vi "IECal-Find Last N.vi"(0 "Data folder":path, 7 "Speaker":string) -> (4 "paths":path[](array[path]), 8 "names":string[](array[string]))   [LabVIEW 2020]
doc: "This helper VI plots all of the in ear calibration files in the current experiment data folder.\n\nKEH 9/10/09"
uses:
  <vilib>/regexp/Match Regular Expression.xnode
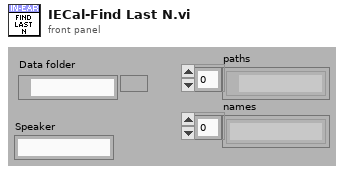
[diagram p1: front panel]
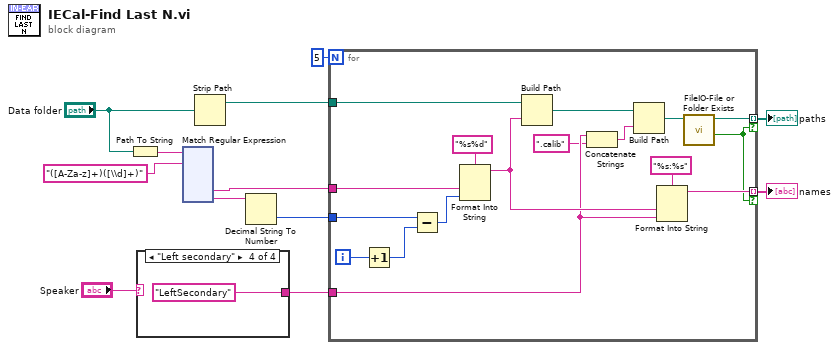
[diagram p0: block diagram]
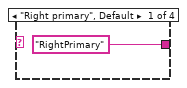
[diagram p2: hidden frame]
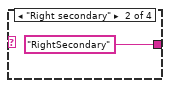
[diagram p3: hidden frame]
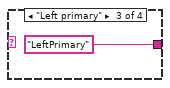
[diagram p4: hidden frame]
diagram:
  n1 = Path To String(path="Data folder") -> (string=w9:string)
  n2 = case shown="\"Left secondary\"" "Speaker" {
    tunnel: ["RightPrimary" "RightSecondary" "LeftPrimary" "LeftSecondary"] -> w3
    frame "Right primary", Default {
    }
    frame "Right secondary" {
    }
    frame "Left primary" {
    }
    frame "Left secondary" {
    }
  }
  n3 = xnode "Match Regular Expression"("input string"=w9, "regular expression"="([A-Za-z]+)([\\d]+)") -> ("submatch 1"=w5:string, "submatch 2"=w7:string)  [unwired: 4 in, 5 out]
  n4 = Strip Path(path="Data folder") -> (stripped path=w4:path)  [unwired: 1 out]
  n5 = Decimal String To Number(string=w7) -> (number=w6:i32)  [unwired: 2 in, 1 out]
  n6 = for {
    N: 5 -> [_]
    tunnel: w6 -> [w32]
    tunnel: w5 -> [w30]
    tunnel: w4 -> [w27]
    tunnel: w3 -> [w19]
    tunnel: [w24] -> w2 mode=indexing if=w20
    tunnel: [w21] -> w1 mode=indexing if=w20
    i -> [w33]
    n7 = Increment(x=w33) -> (x+1=w31:i32)
    n8 = Subtract(x=w32, y=w31) -> (x-y=w29:i32)
    n9 = Format Into String(format string="%s%d", w30, w29) -> (resulting string=w22:string)  [unwired: 2 in, 1 out]
    n10 = Build Path(base path=w27, name or relative path=w22) -> (appended path=w26:path)
    n11 = Concatenate Strings(w19, ".calib" ("string")) -> (w17:string)
    n12 = Build Path(base path=w26, name or relative path=w17) -> (appended path=w25:path)
    n13 = Format Into String(format string="%s:%s", w22, w19) -> (resulting string=w21:string)  [unwired: 2 in, 1 out]
    n14 = call "FileIO-File or Folder Exists.vi"("path"=w25) -> ("Exists?"=w20:bool, "dup path"=w24:path)  [unwired: 7 in, 2 out]
  }
  "paths" <- w2
  "names" <- w1
